vi "Write Data.vi"(8 "error in (no error)":errorcluster, 10 "Data":sgl[][](array[numeric]), 11 "2D Single Data in":refnum<class "2D Single Data.lvclass">) -> (0 "error out":errorcluster, 3 "2D Single Data out":refnum<class "2D Single Data.lvclass">)   [LabVIEW 2014, in "Base Data Class.lvlib" / "2D Single Data.lvclass"]
uses:
  2D Single Data.lvclass
  2D Single Data.lvclass/2D Single Data.ctl
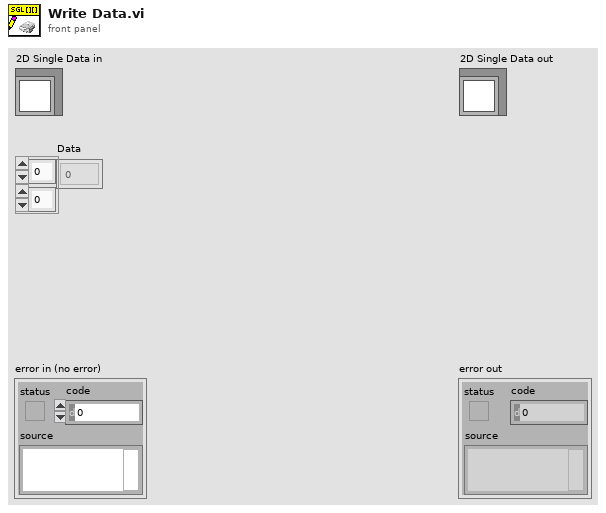
[diagram p1: front panel]
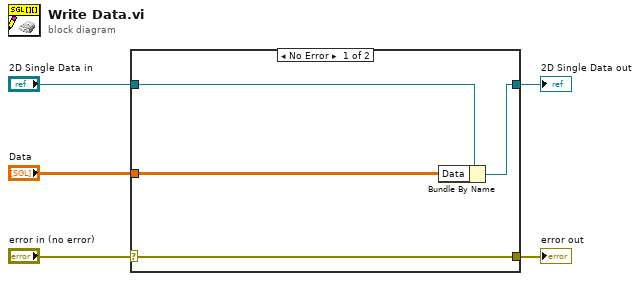
[diagram p0: block diagram]
diagram:
  n1 = case shown="No Error" "error in (no error)" {
    selector: "error in (no error)" -> [w9 w10]
    tunnel: [w9 w10] -> w4
    tunnel: [w7 w11] -> w2
    tunnel: "2D Single Data in" -> [w8 w11]
    tunnel: "Data" -> [w6 _]
    frame No Error {
      n2 = Bundle By Name(cluster=w8, "Data"=w6) -> (w7:refnum<class "2D Single Data.lvclass">)
    }
    frame Error {
    }
  }
  "error out" <- w4
  "2D Single Data out" <- w2
